vi "Read Characters From File with error IO.vi"(0 "file path (dialog if empty)":path, 5 "number of characters (all:-1)":i32=-1, 7 "convert eol? (no:F)":bool, 9 "start of read offset (chars.: 0)":i32, 11 "error in (no error)":errorcluster) -> (4 "new file path (NotAPath if cancelled)":path, 8 "character string":string, 10 "mark after read (chars.)":i32, 13 "EOF?":bool, 15 "error out":errorcluster)   [LabVIEW 2012]
doc: "Reads a specified number of characters from a byte stream file beginning at a specified character offset. The VI opens the file beforehand and closes it afterwards.\n\nfile path is the path name of the file. If file path is empty (default value) or is Not A Path, the VI displays a File dialog box from which you can select a file. Error 43 occurs if the user cancels the dialog. \n\nnumber of character is the maximum number of characters the VI reads. The VI reads fewer characters if it reaches the EOF first. The default value is -1 characters, which means to read the entire file.\n\nstart of read offset is the position in the file, measured in characters (or bytes), at which the VI begins reading.\n\nnew file path is the path of the file from which the VI read data. You can use this output to determine the path of a file that you open using dialog. new file path returns Not A Path if the user selects Cancel from the dialog box.\n\ncharacters string is the data read from the file\n\nmark after read is the location of the file mark after the read; it points to the character in the file following the last character read.\n\nEOF? is TRUE if you attempt to read past the end of file."
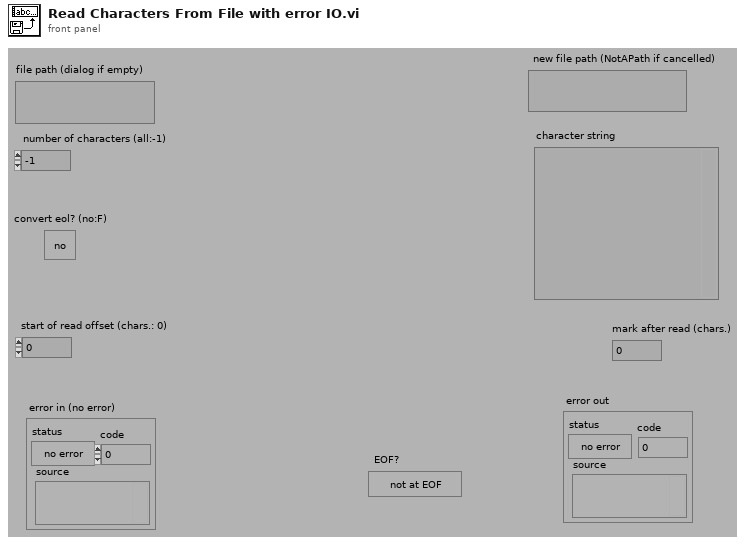
[diagram p1: front panel]
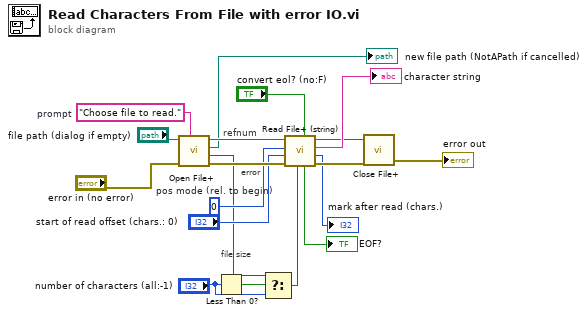
[diagram p0: block diagram]
diagram:
  w16 = i16 0  # pos mode (rel. to begin)
  w11 = "Choose file to read."  # prompt
  # "file size"
  # "error"
  # "refnum"
  n1 = call <vilib>:"Open File+.vi"("prompt"=w11, "error in (not an error)"="error in (no error)", "file path (\" \")"="file path (dialog if empty)") -> ("error out"=w18:errorcluster, "file size (bytes)"=w6:i32, "file path"=→"new file path (NotAPath if cancelled)":path, "refnum"=w9:refnum<file>)  [unwired: 3 in, 2 out]
  n2 = Less Than 0?(x="number of characters (all:-1)") -> (x < 0?=w7:bool)
  n3 = Select(t=w6, s=w7, f="number of characters (all:-1)") -> (s? t:f=w4:i32)
  n4 = call <vilib>:"Read File+ (string).vi"("convert eol? (no:F)"="convert eol? (no:F)", "count"=w4, "error in (no error)"=w18, "pos offset (bytes:0)"="start of read offset (chars.: 0)", "pos mode (rel. to current:2)"=w16, "refnum"=w9) -> ("error out"=w14:errorcluster, "mark after read (bytes)"=→"mark after read (chars.)":i32, "string"=→"character string":string, "dup refnum"=w13:refnum<file>, "EOF?"=→"EOF?":bool)  [unwired: 1 out]
  n5 = call <vilib>:"Close File+.vi"("error in (no error)"=w14, "refnum"=w13) -> ("error out"=→"error out":errorcluster)  [unwired: 5 out]
